vi "202_SetGetParameterArray.vi"() -> ()   [LabVIEW 2009]
uses:
  <instrlib>/Zurich Instruments LabOne/Public/Configure/ziSetValueDoubleArray.vi
  <instrlib>/Zurich Instruments LabOne/Public/Configure/ziGetValueDouble.vi
  <instrlib>/Zurich Instruments LabOne/Zurich Instruments LabOne.lvlib
panel:
  out "Set nodes":string[](array[string])=["sigouts/0/on", "sigouts/0/amplitudes/0", "sigouts/0/range"]
  out "Get values":dbl[](array[numeric])
  out "Connected?":bool
  out "Error Out":errorcluster
  in  "Address":string="DEV"
  # "Set-Get an array of parameters\nThis VI shows how to configure your instrument by assigning multiple values to multiple data server nodes. \n\nSee block diagram for the VI description.\n\nRequirements: Any Zurich Instrument Product\n\nTo run\n1- Type the Instrument ID \n2- Run the VI\n* You can change Node1 and Value1 Set in the back panel to set different nodes \n\nTested Devices:\n- HF2LI\n- UHFLI\n- MFLI\n\n(c) Zurich Instruments.  ALL RIGHTS RESERVED."
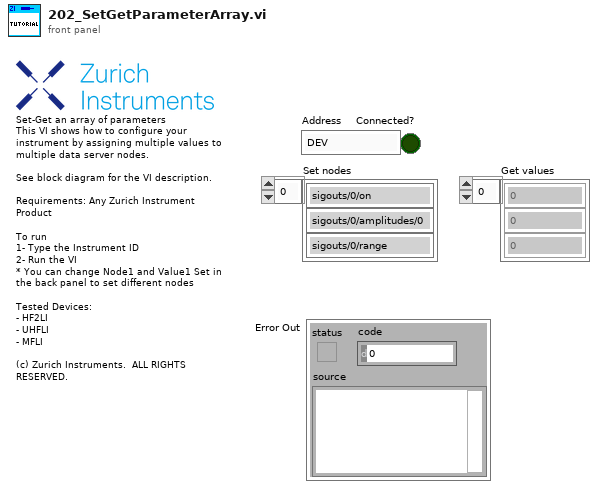
[diagram p1: front panel]
types:
  T1 = typedef "Zurich Instruments LabOne.lvlib/ziTypeHandle.ctl" = cluster{"handleValid":bool, "Conn":u64, "Path Prefix":string, "Handle":u64, "Connected":bool, "Clockbase(s)":dbl}
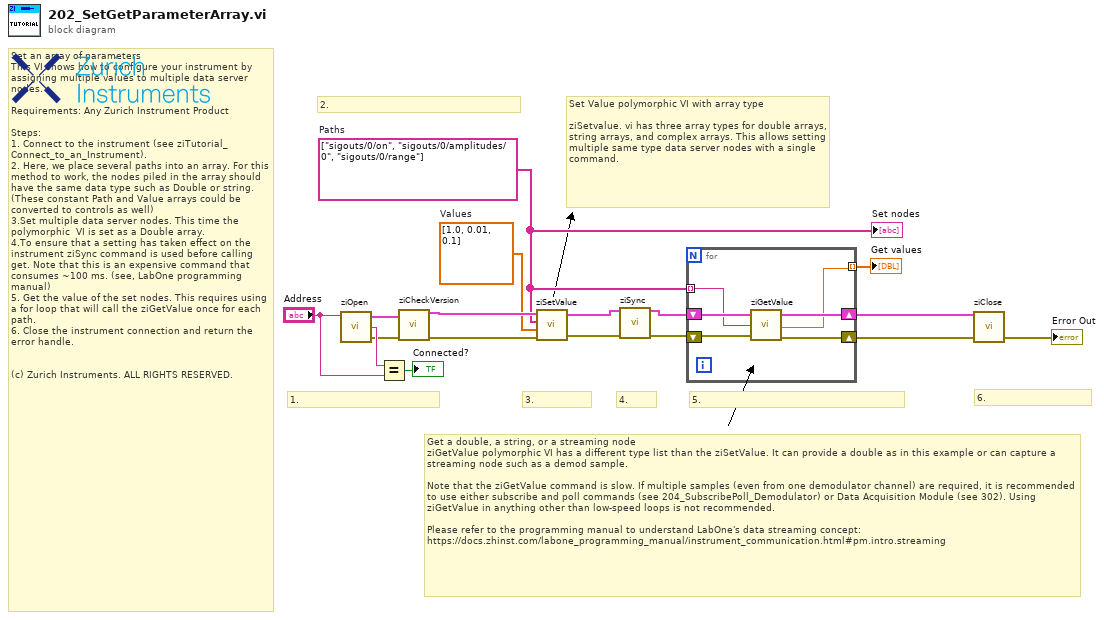
[diagram p0: block diagram]
diagram:
  w3 = dbl[] [1.0, 0.01, 0.1]  # Values
  w2 = string[] ["sigouts/0/on", "sigouts/0/amplitudes/0", "sigouts/0/range"]  # Paths
  # "Get a double, a string, or a streaming node\nziGetValue polymorphic VI has a different type list than the ziSetValue. It can provide a double as in this example or can capture a streaming node such as a demod sample.\n\nNote that the ziGetValue command is slow. If multiple samples (even from one demodulator channel) are required, it is recommended to use either subscribe and poll commands (see 204_SubscribePoll_Demodulator) or Data Acquisition Module (see 302). Using ziGetValue in anything other than low-speed loops is not recommended.\n\nPlease refer to the programming manual to understand LabOne's data streaming concept: \nhttps://docs.zhinst.com/labone_programming_manual/instrument_communication.html#pm.intro.streaming"
  # "2."
  # "Set Value polymorphic VI with array type  \n\nziSetvalue. vi has three array types for double arrays, string arrays, and complex arrays. This allows setting multiple same type data server nodes with a single command."
  # "5."
  # "4."
  # "3."
  # "1."
  # "6."
  # "Set an array of parameters\nThis VI shows how to configure your instrument by assigning multiple values to multiple data server nodes. \n\nRequirements: Any Zurich Instrument Product\n\nSteps:\n1. Connect to the instrument (see ziTutorial_Connect_to_an_Instrument).\n2. Here, we place several paths into an array. For this method to work, the nodes piled in the array should have the same data type such as Double or string. (These constant Path and Value arrays could be converted to controls as well)\n3.Set multiple data server nodes. This time the polymorphic  VI is set as a Double array. \n4.To ensure that a setting has taken effect on the instrument ziSync command is used before calling get. Note that this is an expensive command that consumes ~100 ms. (see, LabOne programming manual)\n5. Get the value of the set nodes. This requires using a for loop that will call the ziGetValue once for each path.\n6. Close the instrument connection and return the error handle.\n\n\n(c) Zurich Instruments. ALL RIGHTS RESERVED."
  n1 = call <instrlib>:"ziOpen.vi"("Address"="Address") -> ("Error Out"=w4:errorcluster, "Selected Device"=w8:string, "HandleOut"=w6:T1)  [unwired: 1 in, 2 out]
  n2 = Equal?(x=w8, y="Address") -> (x = y?=→"Connected?":bool)
  n3 = call <instrlib>:"ziCheckVersion.vi"("Handle In"=w6, "Error In"=w4) -> ("Handle Out"=w10:T1, "Error Out"=w5:errorcluster)  [unwired: 11 in, 1 out]
  n4 = call-poly <instrlib>:"ziSetValue.vi"("Error In"=w5, "Values"=w3, "Paths"=w2, "Handle In"=w10) -> ("Error Out"=w14:errorcluster, "Handle Out"=w12:T1)  [unwired: 1 in]
  n5 = call <instrlib>:"ziSync.vi"("Handle In"=w12, "Error In"=w14) -> ("Handle Out"=w11:T1, "Error Out"=w13:errorcluster)  [unwired: 12 in]
  n6 = for {
    shift-right: [w23] -> w16
    shift-left: w11 -> [w20]
    shift-right: [w22] -> w15
    shift-left: w13 -> [w21]
    tunnel: w2 -> [w19] mode=indexing
    tunnel: [w18] -> w1 mode=indexing
    n7 = call-poly <instrlib>:"ziGetValue.vi"("error in"=w21, "Path"=w19, "Handle in"=w20) -> ("error out"=w22:errorcluster, "Value"=w18:dbl, "Handle out"=w23:T1)
  }
  "Get values" <- w1
  n8 = call <instrlib>:"ziClose.vi"("Error In"=w15, "Handle In"=w16) -> ("Error Out"=→"Error Out":errorcluster)  [unwired: 2 in, 1 out]
  "Set nodes" <- w2
